vi "NIFPGA-MCS.constructor.vi"(0 "name":string, 2 "data in":string, 5 "error in (no error)":errorcluster) -> (14 "i ref out":refnum<vi>, 16 "data out":string, 19 "error out":errorcluster)   [LabVIEW 2014, in "NIFPGA-MCS.lvlib"]
doc: "This is the constructor of a class.\n\nLicense Agreement for this software:\n\nCopyright (C)\nGesellschaft für Schwerionenforschung, GSI\nPlanckstr. 1\n64291 Darmstadt\nGermany\n\nContact: D.Beck@gsi.de \n\nThis program is free software; you can redistribute it and/or modify it under the terms of the \nGNU General Public License as published by the Free Software Foundation; either version 2 of \nthe license, or (at your option) any later version.\n\nThis program is distributed in the hope that it will be useful, but WITHOUT ANY WARRANTY; \nwithout even the implied warranty of MERCHANTABILITY or FITNESS FOR A PARTICULAR PURPOSE. See the GNU General License for more details (http://www.gnu.org).\n\nGesellschaft für Schwerionenforschung, GSI\nPlanckstr. 1, 64291 Darmstadt, Germany\nFor all questions and ideas contact: M.Richter@gsi.de, H.Brand@gsi.de or D.Beck@gsi.de.\nLast update: 16-JUN-2004"
uses:
  NIFPGA-MCS.lvlib
  CS_Core/CSApplicationBaseClasses/DeviceBase/DeviceBase.myEventNames.ctl
  CS_Core/CSApplicationBaseClasses/MCSBase/MCSBase.myEventNames.ctl
  CS_Core/CSSystem/CSSystemLib/CSSystemLib.lvlib
  CS_Core/CSApplicationBaseClasses/MCSBase/MCSBase.lvlib
  CS_Core/CSApplicationBaseClasses/DeviceBase/DeviceBase.lvlib
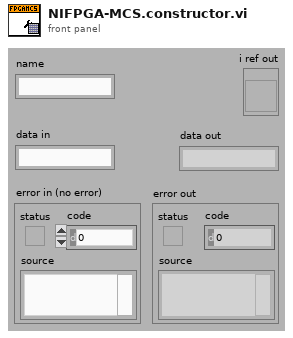
[diagram p1: front panel]
types:
  T1 = enum16{"SetAttribute", "GetAttribute", "CreateAttribute", "DestroyAttribute", "DestroyAllAtributes"}
  T2 = typedef "MCSBase.lvlib/MCSBase.myEventNames.ctl" = enum16{"lvmsg://SetBinWidth", "lvmsg://SetBinsPerRecord", "lvmsg://SetRecordsPerScan", "lvmsg://StartScan", "lvmsg://StopScan", "lvmsg://GetScanStatus", "lvmsg://GetBinData", "lvmsg://GetBinWidth", "lvmsg://GetBinsPerRecord", "lvmsg://GetRecordsPerScan", "lvmsg://SetTriggerLevel", "lvmsg://SetTriggerSlope", "lvmsg://SetDiscLevel", "lvmsg://SetDiscSlope", "lvmsg://GetTriggerLevel", "lvmsg://GetTriggerSlope", "lvmsg://GetDiscLevel", "lvmsg://GetDiscSlope", "lvmsg://ReadData"}
  T3 = typedef "DeviceBase.lvlib/DeviceBase.myEventNames.ctl" = enum16{"lvmsg://Initialize", "lvmsg://Close", "lvmsg://Configure", "lvmsg://Reset", "lvmsg://IDQuery"}
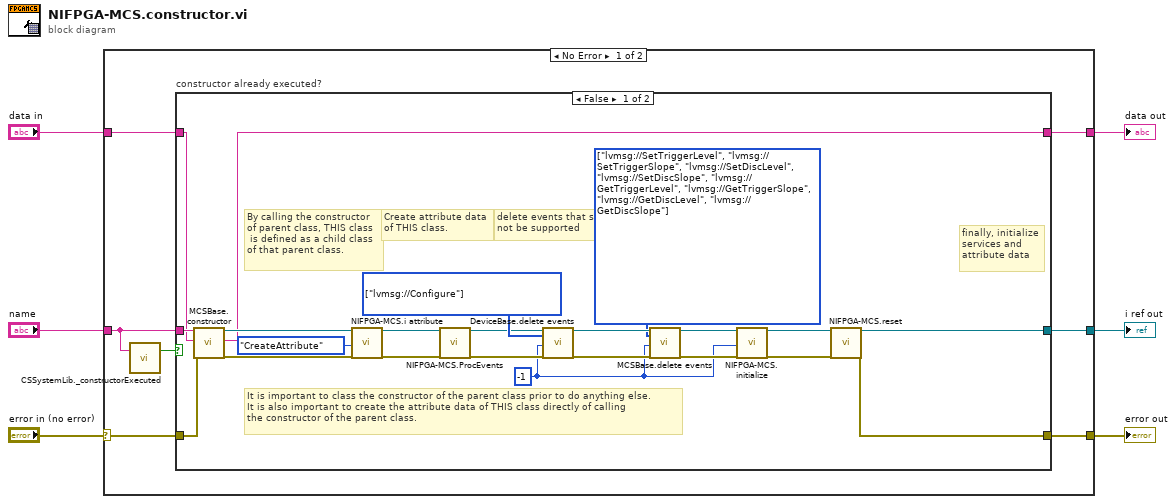
[diagram p0: block diagram]
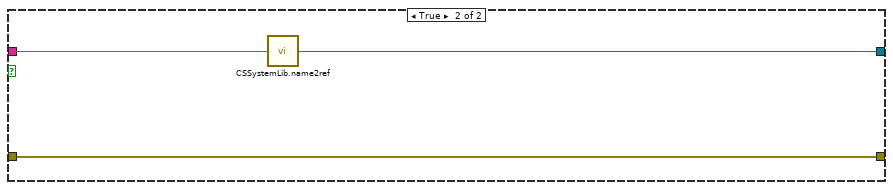
[diagram p2: hidden frame]
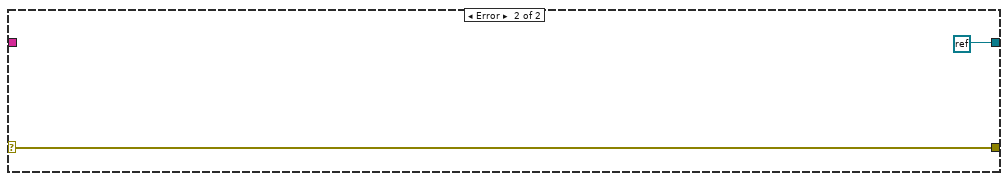
[diagram p3: hidden frame]
diagram:
  n1 = case shown="No Error" "error in (no error)" {
    selector: "error in (no error)" -> [w11 w39]
    tunnel: "name" -> [w10 _]
    tunnel: [w13 refnum<k0> refnum ("Not a Refnum Constant")] -> w5
    tunnel: [w12 w39] -> w4
    tunnel: "data in" -> [w8 _]
    tunnel: [w7 _] -> w1
    frame No Error {
      n2 = call "CSSystemLib._constructorExecuted.vi"("name"=w10) -> ("constructor executed?"=w9:bool)  [unwired: 18 in]
      n3 = case "constructor already executed?" shown="False" w9 {
        tunnel: w10 -> [w32 w38]
        tunnel: [w15 w37] -> w13
        tunnel: [w16 w36] -> w12
        tunnel: w11 -> [w29 w36]
        tunnel: w8 -> [w28 _]
        tunnel: [w14 _] -> w7
        frame False {
          w22 = T2[] [enum."lvmsg://SetTriggerLevel", enum."lvmsg://SetTriggerSlope", enum."lvmsg://SetDiscLevel", enum."lvmsg://SetDiscSlope", enum."lvmsg://GetTriggerLevel", enum."lvmsg://GetTriggerSlope", enum."lvmsg://GetDiscLevel", enum."lvmsg://GetDiscSlope"] items=["lvmsg://SetBinWidth", "lvmsg://SetBinsPerRecord", "lvmsg://SetRecordsPerScan", "lvmsg://StartScan", "lvmsg://StopScan", "lvmsg://GetScanStatus", "lvmsg://GetBinData", "lvmsg://GetBinWidth", "lvmsg://GetBinsPerRecord", "lvmsg://GetRecordsPerScan", "lvmsg://SetTriggerLevel", "lvmsg://SetTriggerSlope", "lvmsg://SetDiscLevel", "lvmsg://SetDiscSlope", "lvmsg://GetTriggerLevel", "lvmsg://GetTriggerSlope", "lvmsg://GetDiscLevel", "lvmsg://GetDiscSlope", "lvmsg://ReadData"] ("events")
          w27 = T3[] [enum."lvmsg://Configure"] items=["lvmsg://Initialize", "lvmsg://Close", "lvmsg://Configure", "lvmsg://Reset", "lvmsg://IDQuery"] ("events")
          w19 = -1 ("ms timeout (10000)")
          # "finally, initialize\nservices and\nattribute data"
          # "delete events that should\nnot be supported"
          # "It is important to class the constructor of the parent class prior to do anything else.\nIt is also important to create the attribute data of THIS class directly of calling\nthe constructor of the parent class."
          # "Create attribute data\nof THIS class."
          # "By calling the constructor\nof parent class, THIS class\n is defined as a child class\nof that parent class."
          n4 = call "MCSBase.constructor.vi"("name"=w32, "data in"=w28, "error in (no error)"=w29) -> ("i ref out"=w35:refnum<vi>, "data out"=w14:string, "error out"=w34:errorcluster)  [unwired: 14 in]
          n5 = call "NIFPGA-MCS.i attribute.vi"("VI Refnum"=w35, "Action"=T1."CreateAttribute", "error in (no error)"=w34) -> ("VI Refnum out"=w31:refnum<vi>, "error out"=w30:errorcluster)  [unwired: 14 in, 1 out]
          n6 = call "NIFPGA-MCS.ProcEvents.vi"("i ref in"=w31, "error in (no error)"=w30) -> ("i ref out"=w26:refnum<vi>, "error out"=w25:errorcluster)  [unwired: 16 in]
          n7 = call "DeviceBase.delete events.vi"("i ref in"=w26, "events"=w27, "ms timeout (10000)"=w19, "error in (no error)"=w25) -> ("i ref out"=w24:refnum<vi>, "error out"=w23:errorcluster)  [unwired: 13 in, 1 out]
          n8 = call "MCSBase.delete events.vi"("i ref in"=w24, "events"=w22, "ms timeout (10000)"=w19, "error in (no error)"=w23) -> ("i ref out"=w21:refnum<vi>, "error out"=w20:errorcluster)  [unwired: 13 in, 1 out]
          n9 = call "NIFPGA-MCS.initialize.vi"("i ref in"=w21, "ms timeout (10000)"=w19, "error in (no error)"=w20) -> ("i ref out"=w18:refnum<vi>, "error out"=w17:errorcluster)  [unwired: 14 in, 1 out]
          n10 = call "NIFPGA-MCS.reset.vi"("i ref in"=w18, "error in (no error)"=w17) -> ("i ref out"=w15:refnum<vi>, "error out"=w16:errorcluster)  [unwired: 16 in]
        }
        frame True {
          n11 = call "CSSystemLib.name2ref.vi"("name"=w38) -> ("obj refnum"=w37:refnum<vi>)
        }
      }
    }
    frame Error {
    }
  }
  "i ref out" <- w5
  "error out" <- w4
  "data out" <- w1
